vi "Add Item to Scene.vi"(8 "error in":errorcluster, 10 "Tree Element":T1, 11 "Scene In":refnum<vi>) -> (0 "error out":errorcluster, 3 "Scene Out":refnum<vi>)   [LabVIEW 2017, in "NI_Robotics_3DKinematics.lvlib"]
uses:
  <vilib>/robotics/Kinematics/Plotting/NI_Robotics_3DKinematics.lvlib
  <vilib>/robotics/Kinematics/Plotting/Tree Element.ctl
  <vilib>/robotics/Kinematics/Plotting/Element Type.ctl
  <vilib>/robotics/Kinematics/Plotting/Joint Type.ctl
  <vilib>/Utility/AngleManip/Degrees to Radians (Scalar DBL).vi
  <vilib>/picture/3D Picture Control/Object/Create Object (name).vi
  <vilib>/picture/3D Picture Control/NI_3D Picture Control.lvlib
  <vilib>/Utility/AngleManip/NI_AngleManipulation.lvlib
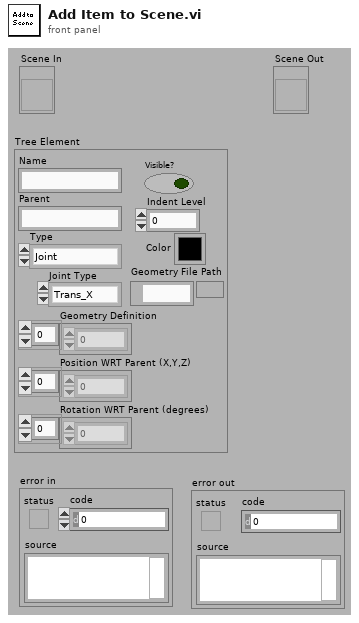
[diagram p1: front panel]
types:
  T1 = typedef "NI_Robotics_3DKinematics.lvlib/Tree Element.ctl" = cluster{"Name":string, "Parent":string, "Type":T2, "Visible?":bool, "Geometry Definition":dbl[], "Position WRT Parent (X,Y,Z)":dbl[], "Rotation WRT Parent (degrees)":dbl[], "Joint Type":T3, "Geometry File Path":path, "Indent Level":i32, "Color":u32}
  T2 = typedef "NI_Robotics_3DKinematics.lvlib/Element Type.ctl" = enum16{"Joint", "Box", "Cylinder", "Cone", "Sphere", "ASE File", "VRML File", "STL File", "Space"}
  T3 = typedef "NI_Robotics_3DKinematics.lvlib/Joint Type.ctl" = enum16{"Trans_X", "Trans_Y", "Trans_Z", "Rot_X", "Rot_Y", "Rot_Z", "None"}
  T4 = cluster{"Position WRT Parent (X,Y,Z)[0]":dbl, "Position WRT Parent (X,Y,Z)[1]":dbl, "Position WRT Parent (X,Y,Z)[2]":dbl}
  T5 = cluster{"Rotation WRT Parent (degrees)[0]":dbl, "Rotation WRT Parent (degrees)[1]":dbl, "Rotation WRT Parent (degrees)[2]":dbl}
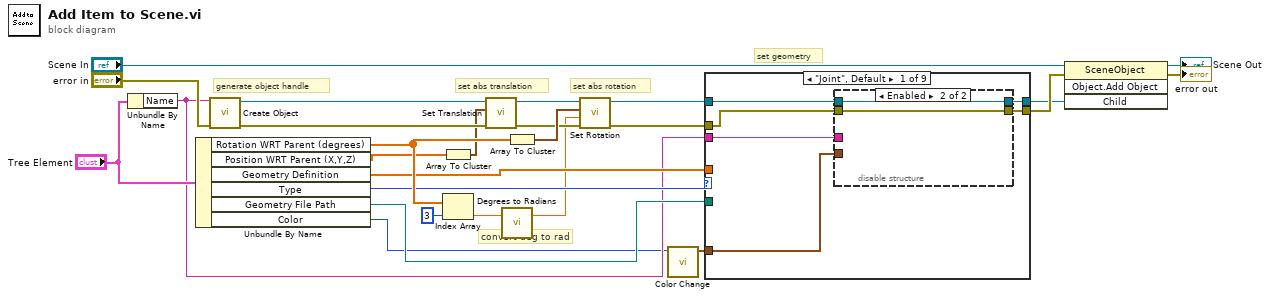
[diagram p0: block diagram]
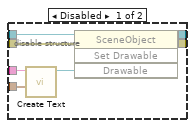
[diagram p2: hidden frame]
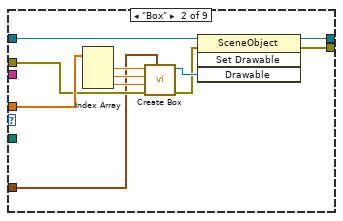
[diagram p3: hidden frame]
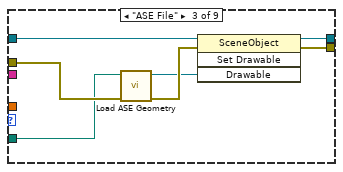
[diagram p4: hidden frame]
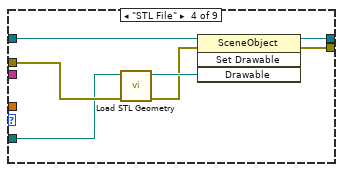
[diagram p5: hidden frame]
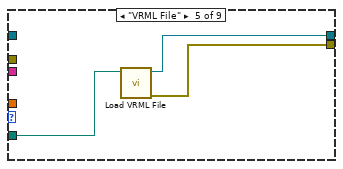
[diagram p6: hidden frame]
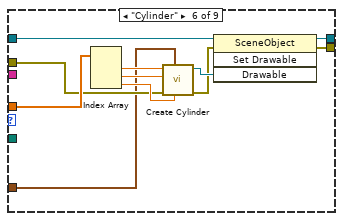
[diagram p7: hidden frame]
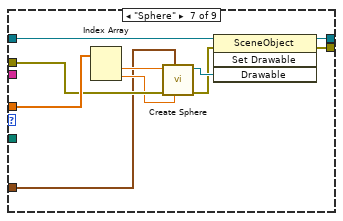
[diagram p8: hidden frame]
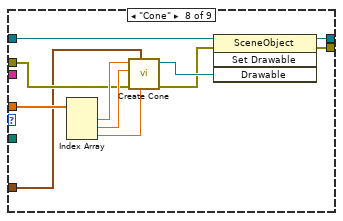
[diagram p9: hidden frame]
diagram:
  # "set abs rotation"
  # "set abs translation"
  # "set geometry"
  # "generate object handle"
  # "convert deg to rad"
  n1 = Unbundle By Name("Tree Element") -> ("Name"=w9:string)
  n2 = Unbundle By Name("Tree Element") -> ("Rotation WRT Parent (degrees)"=w24:dbl[], "Position WRT Parent (X,Y,Z)"=w19:dbl[], "Geometry Definition"=w14:dbl[], "Type"=w12:T2, "Geometry File Path"=w10:path, "Color"=w8:u32)
  n3 = call-poly <vilib>:"Create Object.vi"("error in (no error)"="error in", "Name"=w9) -> ("error out"=w20:errorcluster, "Scene:New Object"=w21:refnum<vi>)  [unwired: 8 in]
  n4 = Array To Cluster(array=w19) -> (cluster=w3:T4)
  n5 = Index Array(array=w24, index=3) -> (element=w2:dbl)
  n6 = call <vilib>:"Set Translation.vi"("error in (no error)"=w20, "Translation"=w3, "Scene Object"=w21) -> ("error out"=w5:errorcluster, "Translated Object"=w4:refnum<vi>)  [unwired: 7 out]
  n7 = call-poly <vilib>:"Degrees to Radians.vi"("angle (deg)"=w2) -> ("angle (rad)"=w1:dbl)  [unwired: 2 in]
  n8 = Array To Cluster(array=w24) -> (cluster=w6:T5)
  n9 = call <vilib>:"Set Rotation.vi"("error in (no error)"=w5, "Angle"=w1, "Axis"=w6, "Scene Object"=w4) -> ("error out"=w23:errorcluster, "Rotated Scene Object"=w22:refnum<vi>)  [unwired: 6 out]
  n10 = call <vilib>:"Color Change.vi"("Color"=w8) -> ("RGBA"=w7:cluster{"R":sgl, "G":sgl, "B":sgl, "A":sgl})  [unwired: 1 in, 9 out]
  n11 = case shown="\"Joint\", Default" w12 {
    tunnel: w22 -> [w30 w52 w53 w66 _ w80 w90 w101 w103]
    tunnel: [w29 w51 w59 w65 w68 w79 w89 w100 w103] -> w13
    tunnel: w14 -> [_ w50 _ _ _ w78 w88 w99 _]
    tunnel: w23 -> [w32 w45 w58 w63 _ w73 w86 w92 w102]
    tunnel: [w28 w43 w56 w61 w67 w71 w84 w94 w102] -> w16
    tunnel: w10 -> [_ _ w55 w60 w69 _ _ _ _]
    tunnel: w9 -> [w31 _ _ _ _ _ _ _ _]
    tunnel: w7 -> [w27 w42 _ _ _ w70 w81 w91 _]
    frame "Joint", Default {
      n12 = disable-structure shown="Enabled" {
        disable-tunnel: w32 -> [w38 w40]
        disable-tunnel: w31 -> [w37 _]
        disable-tunnel: w30 -> [w36 w41]
        disable-tunnel: [w35 w41] -> w29
        disable-tunnel: [w34 w40] -> w28
        disable-tunnel: w27 -> [w33 _]
        frame Disabled {
          n13 = call <vilib>:"Create Text.vi"("Color"=w33, "Text"=w37) -> ("New Text Refnum"=w39:refnum<vi>)  [unwired: 2 in, 7 out]
          n14 = invoke class="SceneObject" method="Set Drawable"(reference=w36, error in=w38, "Drawable"=w39) -> (reference out=w35:refnum<vi>, error out=w34:errorcluster)  [unwired: 1 in, 2 out]
        }
        frame Enabled {
        }
      }
    }
    frame "Box" {
      n15 = Index Array(array=w50) -> (element #1=w49:dbl, element #2=w48:dbl, element #3=w47:dbl)  [unwired: 3 in]
      n16 = call <vilib>:"Create Box.vi"("Color"=w42, "error in (no error)"=w45, "Length Z"=w47, "Length Y"=w48, "Length X"=w49) -> ("error out"=w44:errorcluster, "New Box Refnum"=w46:refnum<vi>)  [unwired: 5 out]
      n17 = invoke class="SceneObject" method="Set Drawable"(reference=w52, error in=w44, "Drawable"=w46) -> (reference out=w51:refnum<vi>, error out=w43:errorcluster)  [unwired: 1 in, 2 out]
    }
    frame "ASE File" {
      n18 = call <vilib>:"Load ASE Geometry.vi"("error in (no error)"=w58, "Model File"=w55) -> ("error out"=w57:errorcluster, "New Mesh Refnum"=w54:refnum<vi>)  [unwired: 2 in, 6 out]
      n19 = invoke class="SceneObject" method="Set Drawable"(reference=w53, error in=w57, "Drawable"=w54) -> (reference out=w59:refnum<vi>, error out=w56:errorcluster)  [unwired: 1 in, 2 out]
    }
    frame "STL File" {
      n20 = call <vilib>:"Load STL Geometry.vi"("error in (no error)"=w63, "Model File"=w60) -> ("error out"=w62:errorcluster, "New Mesh Refnum"=w64:refnum<vi>)  [unwired: 8 out]
      n21 = invoke class="SceneObject" method="Set Drawable"(reference=w66, error in=w62, "Drawable"=w64) -> (reference out=w65:refnum<vi>, error out=w61:errorcluster)  [unwired: 1 in, 2 out]
    }
    frame "VRML File" {
      n22 = call <vilib>:"Load VRML File.vi"("Path"=w69) -> ("error out"=w67:errorcluster, "Scene:Read Scene File"=w68:refnum<vi>)  [unwired: 1 in, 8 out]
    }
    frame "Cylinder" {
      n23 = Index Array(array=w78) -> (element #1=w77:dbl, element #2=w76:dbl, element #3=w75:dbl)  [unwired: 3 in]
      n24 = call <vilib>:"Create Cylinder.vi"("Detail"=w75, "Color"=w70, "error in (no error)"=w73, "Radius"=w76, "Height"=w77) -> ("error out"=w72:errorcluster, "New Cylinder Refnum"=w74:refnum<vi>)  [unwired: 5 out]
      n25 = invoke class="SceneObject" method="Set Drawable"(reference=w80, error in=w72, "Drawable"=w74) -> (reference out=w79:refnum<vi>, error out=w71:errorcluster)  [unwired: 1 in, 2 out]
    }
    frame "Sphere" {
      n26 = Index Array(array=w88) -> (element #1=w83:dbl, element #2=w82:dbl)  [unwired: 2 in]
      n27 = call <vilib>:"Create Sphere.vi"("Detail"=w82, "Color"=w81, "error in (no error)"=w86, "Radius"=w83) -> ("error out"=w85:errorcluster, "New Sphere Refnum"=w87:refnum<vi>)  [unwired: 1 in, 5 out]
      n28 = invoke class="SceneObject" method="Set Drawable"(reference=w90, error in=w85, "Drawable"=w87) -> (reference out=w89:refnum<vi>, error out=w84:errorcluster)  [unwired: 1 in, 2 out]
    }
    frame "Cone" {
      n29 = Index Array(array=w99) -> (element #1=w98:dbl, element #2=w97:dbl, element #3=w96:dbl)  [unwired: 3 in]
      n30 = call <vilib>:"Create Cone.vi"("Detail"=w96, "Color"=w91, "error in (no error)"=w92, "Radius"=w97, "Height"=w98) -> ("error out"=w93:errorcluster, "New Cone Refnum"=w95:refnum<vi>)  [unwired: 5 out]
      n31 = invoke class="SceneObject" method="Set Drawable"(reference=w101, error in=w93, "Drawable"=w95) -> (reference out=w100:refnum<vi>, error out=w94:errorcluster)  [unwired: 1 in, 2 out]
    }
    frame "Space" {
    }
  }
  n32 = invoke class="SceneObject" method="Object.Add Object"(reference="Scene In", error in=w16, "Child"=w13) -> (reference out=→"Scene Out":refnum<vi>, error out=→"error out":errorcluster)  [unwired: 1 in, 2 out]
